vi "PicoScope2000aExampleBlock.vi"() -> ()   [LabVIEW 2020]
panel:
  out "overflow (binary)":i16 format="%06b"
  out "Analog Channels":T1(graph)
  in  "Acquisition Settings":T2={"preTriggerSamples"=0, "postTriggerSamples"=1000, "timebase"=2, "Oversample"=1} {"postTriggerSamples" format="%.6p"; "preTriggerSamples" format="%.6p"}
  in  "Buffer and Transfer Settings":T3={"startIndex"=0, "Samples"=1000, "Down Sample Ratio"=2, "Down-Sample Mode"=0} {"Down-Sample Mode" items=["None"=0, "Aggregate"=1, "Decimate"=2, "Average"=4]}
  in  "Channel B Settings":T4={"Enabled"=FALSE, "Coupling"=1, "Range"=6, "Analogue Offset"=0.0} {"Range" items=["20 mV"=1, "50 mV"=2, "100 mV"=3, "200 mV"=4, "500 mV"=5, "1 V"=6, "2 V"=7, "5 V"=8, "10 V"=9, "20 V"=10]; "Coupling" items=["AC", "DC"]}
  in  "Channel A Settings":T4={"Enabled"=TRUE, "Coupling"=1, "Range"=6, "Analogue Offset"=0.0} {"Range" items=["20 mV"=1, "50 mV"=2, "100 mV"=3, "200 mV"=4, "500 mV"=5, "1 V"=6, "2 V"=7, "5 V"=8, "10 V"=9, "20 V"=10]; "Coupling" items=["AC", "DC"]}
  in  "Trigger Settings":T5={"Trigger Enabled"=FALSE, "Trigger Source"=enum."Channel A", "Trigger Threshold (Volts)"=0.0, "Trigger Direction"=2, "Trigger Delay (samples)"=0, "Auto Trigger Time (ms)"=1000} {"Trigger Direction" items=["Rising"=2, "Falling"=3]}
  out "Properties Panel":T6 {"Max Total Capture Time Available (sec)" format="%.3p"; "Sample Frequency" format="%_5p"; "Sample Interval" format="%_5p"; "Max Samples Available" format="%.3p"; "Total Capture Time (sec)" format="%.3p"}
  in  "stop":bool
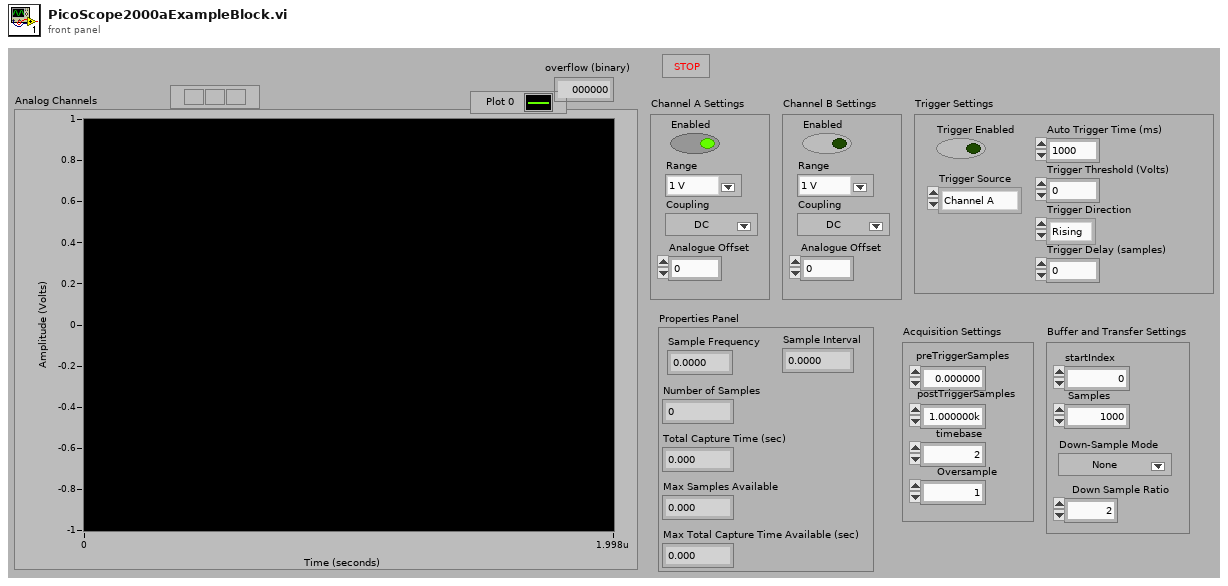
[diagram p1: front panel]
types:
  T1 = cluster{i32, "Sample Internal":sgl, "Data":dbl[]}[]
  T2 = cluster{"preTriggerSamples":u32, "postTriggerSamples":u32, "timebase":u32, "Oversample":i16}
  T3 = cluster{"startIndex":u32, "Samples":u32, "Down Sample Ratio":u32, "Down-Sample Mode":u32}
  T4 = cluster{"Enabled":bool, "Coupling":i16, "Range":u16, "Analogue Offset":sgl}
  T5 = cluster{"Trigger Enabled":bool, "Trigger Source":enum16{"Channel A", "Channel B", "Channel C", "Channel D", "Ext."}, "Trigger Threshold (Volts)":dbl, "Trigger Direction":u16, "Trigger Delay (samples)":u32, "Auto Trigger Time (ms)":i16}
  T6 = cluster{"Sample Frequency":sgl, "Sample Interval":sgl, "Max Samples Available":i32, "Number of Samples":u32, "Total Capture Time (sec) ":sgl, "Max Total Capture Time Available (sec)":sgl}
  T7 = cluster{"Driver Version":string, "USB Version":string, "Hardware":string, "Variant":string, "Batch and Serial":string, "Cal Date":string, "Kernel Version":string, "Digital HW Version":string, "Analogue HW Version":string, "Firmware 1":string, "Firmware 2":string, "MSO":bool, "Number of Channels":i16}
  T8 = cluster{"preTriggerSamples":u32, "postTriggerSamples":u32, "timebase":u32, i32, u32, "Oversample":i16}
  T9 = cluster{"Sample Frequency":sgl, "Sample Internal":sgl, "Max Samples Available":i32, "Number of Samples":u32, "Total Capture Time (sec) ":sgl, "Max Total Capture Time Available (sec)":sgl}
  T10 = cluster{"Channel D Buffer":i16[], "Channel C Buffer":i16[], "Channel B Buffer":i16[], "Channel A Buffer":i16[], "Port 0  Buffer ":i16[], "Port 1 Buffer ":i16[]}
  T11 = cluster{i32, "Sample Internal":sgl, "Data":dbl[]}
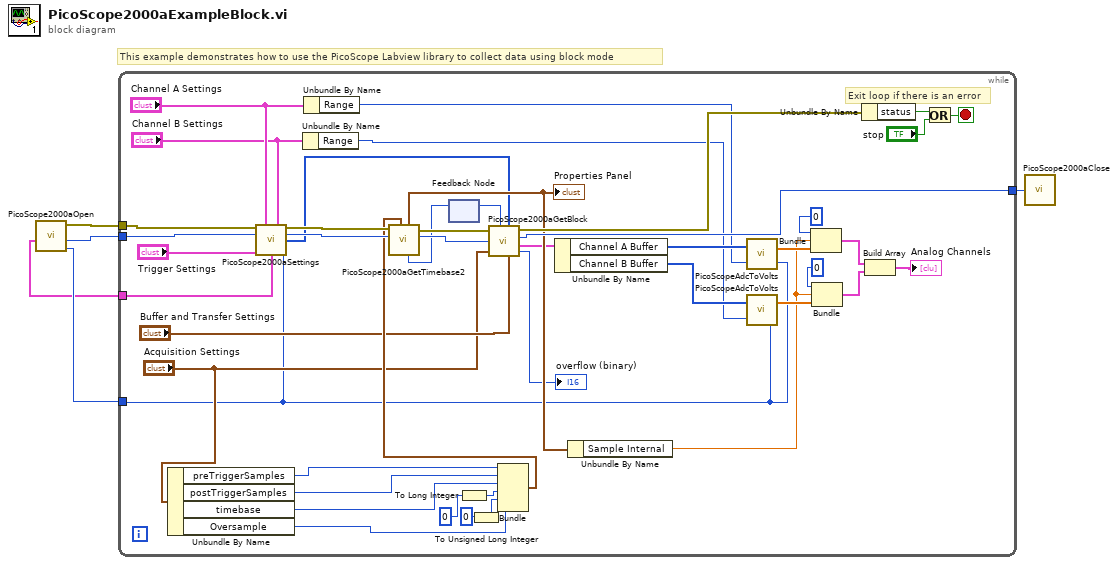
[diagram p0: block diagram]
diagram:
  # "This example demonstrates how to use the PicoScope Labview library to collect data using block mode"
  n1 = call "PicoScope2000aOpen.vi"() -> ("Max Adc value"=w2:i16, "handle"=w4:i16, "error out"=w5:errorcluster, "Device Info"=w1:T7)  [unwired: 4 in]
  n2 = while {
    tunnel: w4 -> [w48]
    tunnel: w5 -> [w47]
    tunnel: [w46] -> w3
    tunnel: w2 -> [w6]
    tunnel: w1 -> [w27]
    stop <- w50 stop-if-true
    # "Exit loop if there is an error"
    n3 = Unbundle By Name("Acquisition Settings") -> ("preTriggerSamples"=w21:u32, "postTriggerSamples"=w20:u32, "timebase"=w19:u32, "Oversample"=w17:i16)
    n4 = call "PicoScope2000aSettings.vi"("error in"=w47, "Channel A Settings"="Channel A Settings", "Channel B Settings"="Channel B Settings", "handle in"=w48, "Trigger Settings"="Trigger Settings", "Device Info"=w27, "Max_adc"=w6) -> ("error out"=w39:errorcluster, "handle out"=w40:i16, "Enabled Array"=w22:i16[])  [unwired: 6 in]
    n5 = Unbundle By Name("Channel B Settings") -> ("Range"=w23:u16)
    n6 = Unbundle By Name("Channel A Settings") -> ("Range"=w24:u16)
    n7 = feedback #1() -> (w37:u64)  [unwired: 1 in]
    n8 = To Long Integer(number=0) -> (32bit integer=w15:i32)
    n9 = To Unsigned Long Integer(number=0) -> (unsigned 32bit integer=w13:u32)
    n10 = Bundle("preTriggerSamples"=w21, "postTriggerSamples"=w20, "timebase"=w19, w15, w13, "Oversample"=w17) -> (w18:T8)  [unwired: 1 in]
    n11 = call "PicoScope2000aGetTimebase2.vi"("Number of Samples"=w37, "Acquisition Settings"=w18, "handle in"=w40, "error in (no error)"=w39) -> ("handle out"=w41:i16, "error out"=w42:errorcluster, "Properties Panel"=w32:T9)  [unwired: 5 in]
    "Properties Panel" <- w32
    n12 = call "PicoScope2000aGetBlock.vi"("error in"=w42, "handle in"=w41, "Acquisition Settings"="Acquisition Settings", "enabled array"=w22, "Buffer and Transfer Settings"="Buffer and Transfer Settings") -> ("noOfSamples"=w38:u64, "overflow (binary)"=→"overflow (binary)":i16, "error out"=w45:errorcluster, "handle out"=w46:i16, "Buffers (Max or non-aggregated)"=w31:T10)  [unwired: 1 out]
    n13 = feedback-in #1(w38) -> ()
    n14 = Unbundle By Name(w31) -> ("Channel A Buffer"=w43:i16[], "Channel B Buffer"=w26:i16[])
    n15 = Unbundle By Name(w32) -> ("Sample Internal"=w28:sgl)
    n16 = call "PicoScopeAdcToVolts.vi"("Max_adc"=w6, "Range Index"=w24, "Data"=w43) -> ("Data"=w33:dbl[])
    n17 = call "PicoScopeAdcToVolts.vi"("Max_adc"=w6, "Range Index"=w23, "Data"=w26) -> ("Data"=w30:dbl[])
    n18 = Bundle(0, "Sample Internal"=w28, "Data"=w33) -> (w9:T11)  [unwired: 1 in]
    n19 = Bundle(0, "Sample Internal"=w28, "Data"=w30) -> (w8:T11)  [unwired: 1 in]
    n20 = Unbundle By Name(w45) -> ("status"=w44:bool)
    n21 = Build Array(w9, w8) -> (→"Analog Channels":T1)
    n22 = Or(x=w44, y="stop") -> (x .or. y?=w50:bool)
  }
  n23 = call "PicoScope2000aClose.vi"("handle"=w3) -> ()
